vi "MARS_Scan_Read_TDMS_Properties.vi"(8 "Active Meas.":i32, 11 "Listbox":i32[](array[numeric])) -> ()   [LabVIEW 2015]
uses:
  ESA_Data_Analysis_Global_VIs.vi
  MARS_Scan_Data_Analysis_global.vi
  MARS_Global_var.vi
panel:
  out "subarray":string[](array[string])
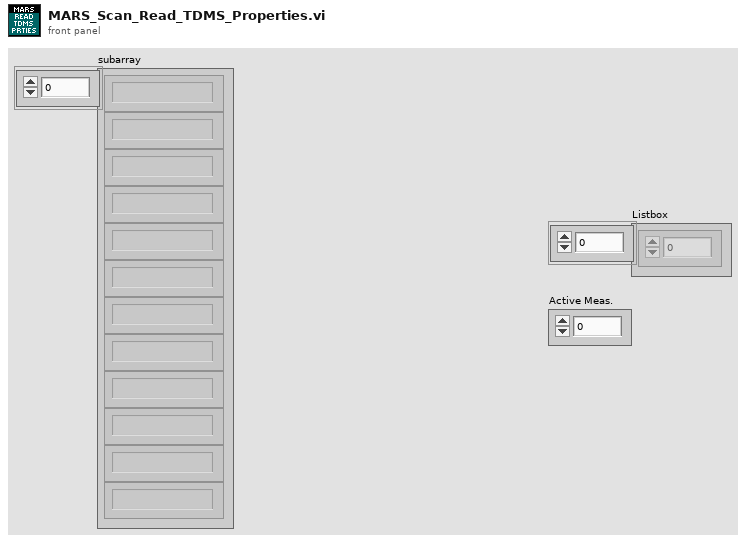
[diagram p1: front panel]
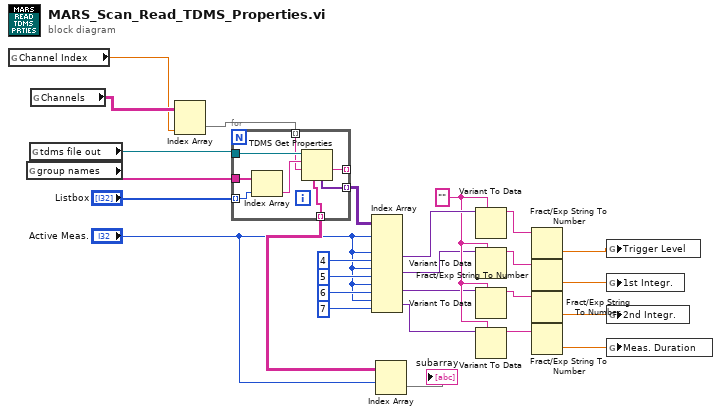
[diagram p0: block diagram]
diagram:
  w11 = ""
  n1 = global read "MARS_Scan_Data_Analysis_global.vi" "Channel Index"() -> (w21:dbl)
  n2 = global read "ESA_Data_Analysis_Global_VIs.vi" "group names"() -> (w24:string[])
  n3 = global read "ESA_Data_Analysis_Global_VIs.vi" "tdms file out"() -> (w25:refnum<k34>)
  n4 = global read "MARS_Scan_Data_Analysis_global.vi" "Channels"() -> (w23:string[][])
  n5 = Index Array(array=w23, index (col)=w21) -> (element=w22:string[])  [unwired: 1 in]
  n6 = for {
    tunnel: w25 -> [w35]
    tunnel: "Listbox" -> [w33] mode=indexing
    tunnel: w24 -> [w34]
    tunnel: [w31] -> w27 mode=indexing
    tunnel: [w30] -> _ mode=indexing
    tunnel: w22 -> [w29] mode=indexing
    tunnel: [w28] -> w3 mode=indexing
    n7 = Index Array(array=w34, index=w33) -> (element=w32:string)
    n8 = TDMS Get Properties(9:w29, 10:w32, 11:w35) -> (1:w30:string, 4:w31:variant[], 6:w28:string[])  [unwired: 3 in, 3 out]
  }
  n9 = Index Array(array=w27, index (row) #1="Active Meas.", index (row) #2="Active Meas.", index (col) #2=4 ("disabled index (col)"), index (row) #3="Active Meas.", index (col) #3=5 ("disabled index (col)"), index (row) #4="Active Meas.", index (col) #4=6 ("disabled index (col)"), index (row) #5="Active Meas.", index (col) #5=7 ("disabled index (col)")) -> (element #2=w12:variant, element #3=w10:variant, element #4=w9:variant, element #5=w8:variant)  [unwired: 1 in, 1 out]
  n10 = Index Array(array=w3, index (row)="Active Meas.") -> (element=→"subarray":string[])  [unwired: 1 in]
  n11 = Variant To Data(type=w11, Variant=w12) -> (data=w7:string)  [unwired: 1 in, 1 out]
  n12 = Variant To Data(type=w11, Variant=w10) -> (data=w6:string)  [unwired: 1 in, 1 out]
  n13 = Variant To Data(type=w11, Variant=w9) -> (data=w5:string)  [unwired: 1 in, 1 out]
  n14 = Variant To Data(type=w11, Variant=w8) -> (data=w4:string)  [unwired: 1 in, 1 out]
  n15 = Fract/Exp String To Number(string=w7) -> (number=w13:dbl)  [unwired: 3 in, 1 out]
  n16 = Fract/Exp String To Number(string=w6) -> (number=w14:dbl)  [unwired: 3 in, 1 out]
  n17 = Fract/Exp String To Number(string=w5) -> (number=w15:dbl)  [unwired: 3 in, 1 out]
  n18 = Fract/Exp String To Number(string=w4) -> (number=w16:dbl)  [unwired: 3 in, 1 out]
  n19 = global write "MARS_Global_var.vi" "Trigger Level"(w13) -> ()
  n20 = global write "MARS_Global_var.vi" "1st Integr."(w14) -> ()
  n21 = global write "MARS_Global_var.vi" "2nd Integr."(w15) -> ()
  n22 = global write "MARS_Global_var.vi" "Meas. Duration"(w16) -> ()
